vi "Scale Raw Data.vi"(7 "Waveform in":waveform(sgl)) -> (8 "Waveform out":waveform(sgl))   [LabVIEW 2014]
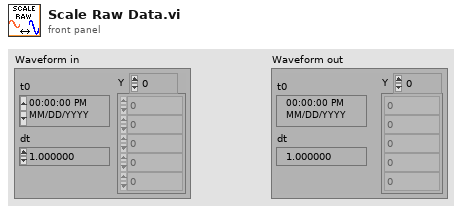
[diagram p1: front panel]
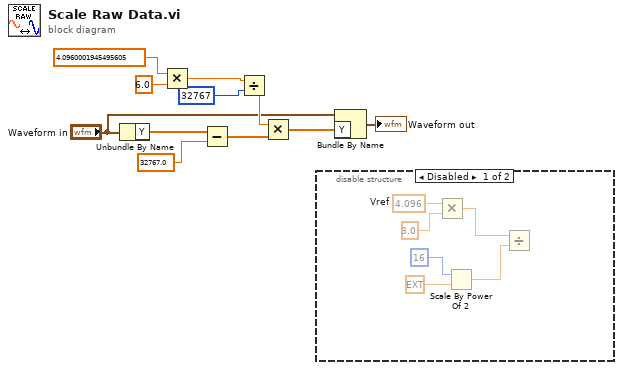
[diagram p0: block diagram]
diagram:
  n1 = Unbundle By Name("Waveform in") -> ("Y"=w7:sgl[])
  n2 = Multiply(x=sgl 4.096, y=sgl 6.0) -> (x*y=w8:sgl)
  n3 = Subtract(x=w7, y=sgl 32767.0 ("x")) -> (x-y=w5:sgl[])
  n4 = Divide(x=w8, y=32767) -> (x/y=w4:sgl)
  n5 = Multiply(x=w4, y=w5) -> (x*y=w2:sgl[])
  n6 = disable-structure shown="Disabled" {
    frame Disabled {
      w15 = 4.096  # Vref
      n7 = Multiply(x=w15, y=3.0) -> (x*y=w13:dbl)
      n8 = Scale By Power Of 2(n=i16 16, x=ext 1.0) -> (x*2^n=w12:ext)
      n9 = Divide(x=w13, y=w12) -> ()  [unwired: 1 out]
    }
    frame Enabled {
    }
  }
  n10 = Bundle By Name(cluster="Waveform in", "Y"=w2) -> (→"Waveform out":waveform(sgl))
